vi "ServiceWatchDog.vi"(8 "error in (no error)":errorcluster, 11 "NHRGridSim in":refnum<class "NHRGridSim.lvclass">) -> (0 "error out":errorcluster, 3 "NHRGridSim out":refnum<class "NHRGridSim.lvclass">)   [LabVIEW 2018, in "AcPwrPlugins.lvlib" / "NHRGridSim.lvclass"]
doc: "This VI send information to the instrument in order to service the robust watch dog setting."
uses:
  NHRGridSim.lvclass
  <instrlib>/NH Research 9400 Series/NH Research 9400 Series.lvlib
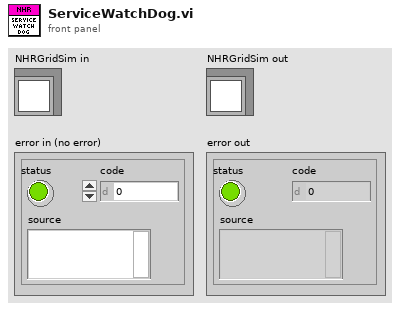
[diagram p1: front panel]
types:
  T1 = typedef "AcPwrPlugins.lvlib/NHRGridSim.lvclass/NHRGrid_Settings.ctl" = cluster{"MeasName":string, "Hardware":T2}
  T2 = typedef "AcPwrPlugins.lvlib/NHRGridSim.lvclass/NHRGrid_Hardware.ctl" = cluster{"Handle":string, "Reset":bool, "Mode":T3, "ID Query":bool, "Logical Instrument":T4}
  T3 = typedef "AcPwrPlugins.lvlib/NHRGridSim.lvclass/NHRGrid_Modes.ctl" = u8
  T4 = typedef "AcPwrPlugins.lvlib/NHRGridSim.lvclass/NHRGrid_Logical_Instrument.ctl" = cluster{"Name":string, "Vout (V)":dbl, "I limit (A)":dbl, "P limit (W)":dbl, "FreqOut (Hz)":dbl, "Ranges":cluster{"Voltage (V)":u16, "Current (A)":u16}, "Configure Instrument":u16, "Aperture (cycles)":i32, "AC Wave Shape":u16, "VType":string, "IType":string, "Phases":T5, "Slew Rates":T6, "Safety Trips":T7}[]
  T5 = typedef "AcPwrPlugins.lvlib/NHRGridSim.lvclass/NHRGrid_Phases.ctl" = cluster{"A-Volts (V)":dbl, "B-Volts (V)":dbl, "C-Volts (V)":dbl, "A-Curr (A)":dbl, "B-Curr (A)":dbl, "C-Curr (A)":dbl, "A-Power (W)":dbl, "B-Power (W)":dbl, "C-Power (W)":dbl, "Change at (Deg)":dbl, "B-Angle (Deg)":dbl, "C-Angle (Deg)":dbl}
  T6 = typedef "AcPwrPlugins.lvlib/NHRGridSim.lvclass/NHRGrid_SlewRates.ctl" = cluster{"Vmax (V/s)":dbl, "Vmin (V/s)":dbl, "Imax (A/s)":dbl, "Imin (A/s)":dbl, "Pmax (W/s)":dbl, "Pmin (W/s)":dbl, "Freq Max (Hz/s)":dbl, "Freq Min (Hz/s)":dbl, "Phase Angle Max (Deg/s)":dbl, "Phase Angle Min (Deg/s)":dbl}
  T7 = typedef "AcPwrPlugins.lvlib/NHRGridSim.lvclass/NHRGrid_SafetyTrips.ctl" = cluster{"Vmax (V)":dbl, "Vmin (V)":dbl, "Vmax Time (s)":dbl, "Vmin Time (s)":dbl, "Imax Source (A)":dbl, "Imax Sink (A)":dbl, "Imax Source Time (s)":dbl, "Imax Sink Time (s)":dbl, "Pmax Source (W)":dbl, "Pmax Sink (W)":dbl, "Pmax Source Time (s)":dbl, "Pmax Sink Time (s)":dbl, "Absolute Volt Peak":dbl, "Enable Volt Peak":bool, "Absolute Curr Peak":dbl, "Enable Curr Peak":bool}
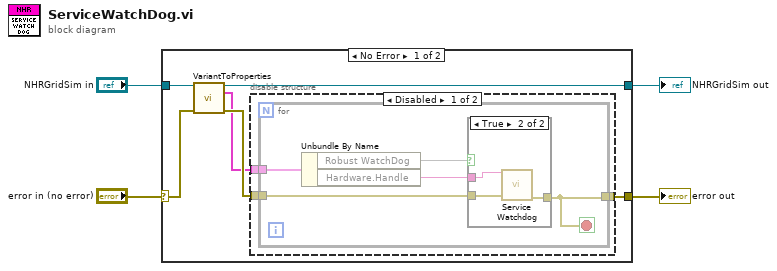
[diagram p0: block diagram]
diagram:
  n1 = case shown="No Error" "error in (no error)" {
    selector: "error in (no error)" -> [w9 w24]
    tunnel: [w6 w24] -> w3
    tunnel: [w8 w23] -> w2
    tunnel: "NHRGridSim in" -> [w10 w23]
    frame No Error {
      n2 = call "VariantToProperties.vi"("NHRGridSim in"=w10, "error in (no error)"=w9) -> ("NHRGridSim out"=w8:refnum<class "NHRGridSim.lvclass">, "Device(s)Settings"=w5:T1, "error out"=w7:errorcluster)  [unwired: 8 in, 3 out]
      n3 = disable-structure shown="Disabled" {
        disable-tunnel: w7 -> [w13 _]
        disable-tunnel: [w12 _] -> w6
        disable-tunnel: w5 -> [w11 _]
        frame Disabled {
          n4 = for {
            tunnel: w11 -> [w18]
            tunnel: w13 -> [w17]
            tunnel: [w16] -> w12
            stop <- w16 stop-if-true
            n5 = Unbundle By Name(w18) -> ("Robust WatchDog"=w15, "Hardware.Handle"=w14:string)
            n6 = case shown="True" w15 {
              tunnel: w14 -> [_ w21]
              tunnel: w17 -> [w19 w22]
              tunnel: [w19 w20] -> w16
              frame False {
              }
              frame True {
                n7 = call <instrlib>:"Service Watchdog.vi"("VISA resource name"=w21, "error in (no error)"=w22) -> ("error out"=w20:errorcluster)  [unwired: 12 in, 1 out]
              }
            }
          }
        }
        frame Enabled {
        }
      }
    }
    frame Error {
    }
  }
  "error out" <- w3
  "NHRGridSim out" <- w2
